vi "Timer FGV.vi"(9 "目标时间(s)":dbl, 11 "定时器命令":T1) -> (1 "已用时间":dbl, 2 "完成？":bool)   [LabVIEW 2012]
doc: "该VI属于功能全局变量，该变量可用于保存将“开始”命令发送至VI后的已使用时间。"
uses:
  TimerCommands.ctl
panel:
  # "输入"
  # "输出"
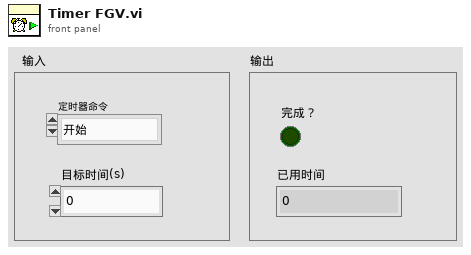
[diagram p1: front panel]
types:
  T1 = typedef "TimerCommands.ctl" = enum16{"开始", "检查时间"}
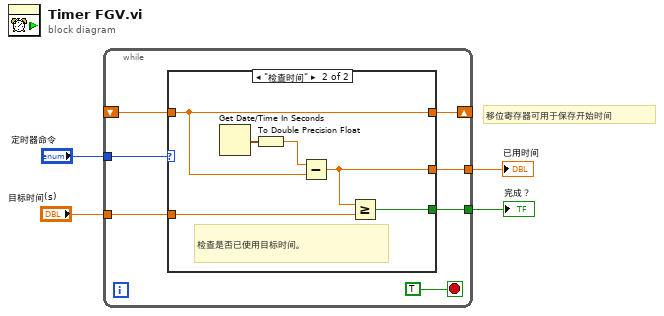
[diagram p0: block diagram]
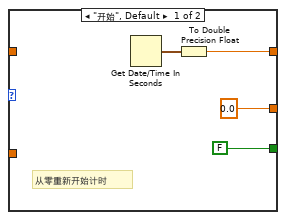
[diagram p2: hidden frame]
diagram:
  # "移位寄存器可用于保存开始时间"
  n1 = while {
    tunnel: "定时器命令" -> [w11]
    shift-right: [w10] -> _
    shift-left: _ -> [w9]
    tunnel: [w8] -> w3
    tunnel: [w7] -> w2
    tunnel: "目标时间(s)" -> [w6]
    stop <- TRUE stop-if-true
    n2 = case shown="\"检查时间\"" w11 {
      tunnel: [w14 w19] -> w10
      tunnel: w9 -> [_ w19]
      tunnel: [0.0 ("双精度浮点数") w18] -> w8
      tunnel: [FALSE w17] -> w7
      tunnel: w6 -> [_ w16]
      frame "开始", Default {
        # "从零重新开始计时"
        n3 = Get Date/Time In Seconds ("获取日期/时间（秒）")() -> (seconds since 1Jan1904=w15:timestamp)
        n4 = To Double Precision Float ("转换为双精度浮点数")(number=w15) -> (double precision float=w14:dbl)
      }
      frame "检查时间" {
        # "检查是否已使用目标时间。"
        n5 = Get Date/Time In Seconds ("获取日期/时间（秒）")() -> (seconds since 1Jan1904=w21:timestamp)
        n6 = To Double Precision Float ("转换为双精度浮点数")(number=w21) -> (double precision float=w20:dbl)
        n7 = Subtract ("减")(x=w20, y=w19) -> (x-y=w18:dbl)
        n8 = Greater Or Equal? ("大于等于？")(x=w18, y=w16) -> (x >= y?=w17:bool)
      }
    }
  }
  "已用时间" <- w3
  "完成？" <- w2
